vi "FRCts20_WebMethods_Comment_PVT_bug.vi"(9 "comment":string, 10 "request":string, 11 "httpRequestID":u32) -> ()   [LabVIEW 2014, in "FRCts20_WebMethods.lvlib"]
uses:
  FRCts20_WebMethods.lvlib
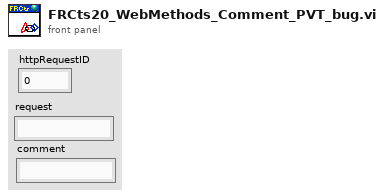
[diagram p1: front panel]
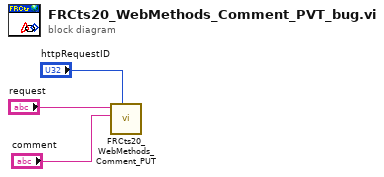
[diagram p0: block diagram]
diagram:
  n1 = call "FRCts20_WebMethods_Comment_PUT.vi"("httpRequestID"="httpRequestID", "comment"="comment", "request"="request") -> ()  [unwired: 9 in]
